vi "Start.vi"(8 "Error In":errorcluster, 11 "Communicator in":refnum<class "Communicator.lvclass">) -> (0 "Error Out":errorcluster, 3 "Communicator out":refnum<class "Communicator.lvclass">)   [LabVIEW 2019, in "Communicator.lvclass"]
uses:
  Communicator.lvclass
  Interfaces/IRunnable/IRunnable.lvclass
  Communicator Worker/Communicator Worker/Communicator Worker.lvclass
  Interfaces/ICommunicate/ICommunicate.lvclass
  Interfaces/IConfigure/IConfigure.lvclass
  Interfaces/IConfiguration/IConfiguration.lvclass
  Communicator.lvclass/Communicator.ctl
  <vilib>/ActorFramework/Actor/Actor.lvclass
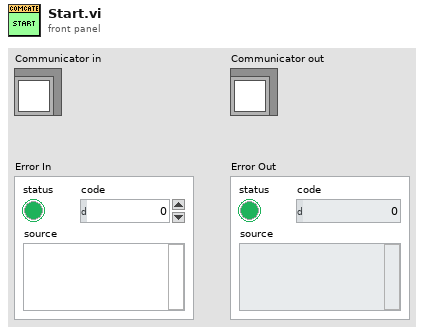
[diagram p1: front panel]
types:
  T1 = typedef "Communicator.lvclass/ObjectAttributes.ctl" = cluster{"IConfigure":refnum<class "IConfigure.lvclass">, "Worker Enqueuer":refnum<class "Message Enqueuer.lvclass">, "Start Counter":i32, "Msg Sent":refnum<user-event>}
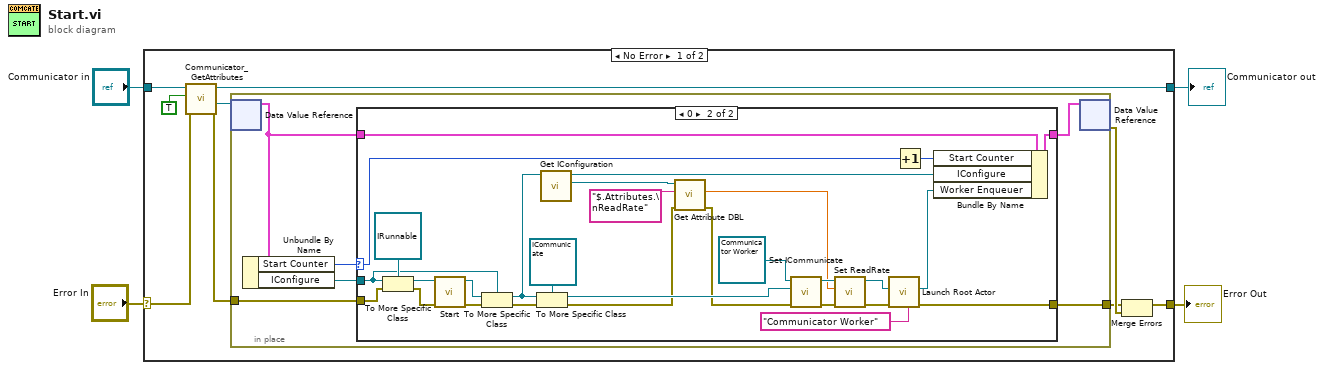
[diagram p0: block diagram]
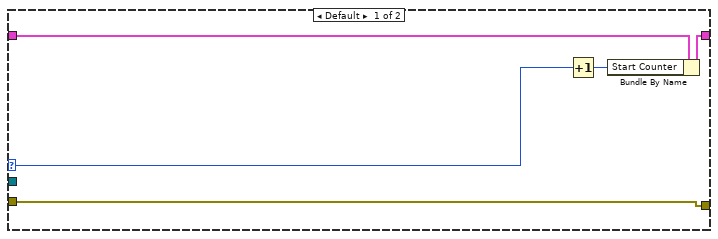
[diagram p2: hidden frame]
diagram:
  n1 = case shown="No Error" "Error In" {
    selector: "Error In" -> [w12 w53]
    tunnel: [w9 w53] -> w3
    tunnel: [w10 w52] -> w1
    tunnel: "Communicator in" -> [w13 w52]
    frame No Error {
      n2 = call "Communicator_GetAttributes.vi"("Error In"=w12, "OnlyGetDvrReference(False)"=TRUE, "Communicator in"=w13) -> ("Error Out"=w6:errorcluster, "DataRef"=w8:refnum<data-value>, "Communicator out"=w10:refnum<class "Communicator.lvclass">)  [unwired: 5 in, 1 out]
      n3 = in-place {
        in-place-border: w6 -> [w17]
        in-place-border: [w16] -> w5
        n4 = in-place-dvr #1(w8) -> (w18:T1)  [unwired: 1 out]
        n5 = Unbundle By Name(w18) -> ("Start Counter"=w14:i32, "IConfigure"=w15:refnum<class "IConfigure.lvclass">)
        n6 = case shown="0" w14 {
          selector: w14 -> [w22 w26]
          tunnel: [w21 w51] -> w19
          tunnel: w18 -> [w23 w50]
          tunnel: w17 -> [w24 w45]
          tunnel: [w24 w44] -> w16
          tunnel: w15 -> [_ w35]
          frame Default {
            n7 = Increment(x=w22) -> (x+1=w20:i32)
            n8 = Bundle By Name(cluster=w23, "Start Counter"=w20) -> (w21:T1)
          }
          frame 0 {
            n9 = To More Specific Class(target class=refnum<class "IRunnable.lvclass"> refnum ("IRunnable.lvclass"), reference=w35, error in=w45) -> (specific class reference=w48:refnum<class "IRunnable.lvclass">, error out=w47:errorcluster)
            n10 = call-dynamic "Start.vi"("error in"=w47, "IRunnable in"=w48) -> ("error out"=w46:errorcluster, "IRunnable out"=w36:refnum<class "IRunnable.lvclass">)  [unwired: 8 in]
            n11 = To More Specific Class(target class=w35, reference=w36, error in=w46) -> (specific class reference=w34:refnum<class "IConfigure.lvclass">, error out=w37:errorcluster)
            n12 = To More Specific Class(target class=refnum<class "ICommunicate.lvclass"> refnum ("ICommunicate.lvclass"), reference=w34, error in=w37) -> (specific class reference=w32:refnum<class "ICommunicate.lvclass">, error out=w29:errorcluster)
            n13 = call-dynamic "Get IConfiguration.vi"("IConfigure in"=w34) -> ("IConfiguration"=w31:refnum<class "IConfiguration.lvclass">, "IConfigure out"=w33:refnum<class "IConfigure.lvclass">)  [unwired: 9 in]
            n14 = call-dynamic "Get Attribute DBL.vi"("error in"=w29, "Attribute"="$.Attributes.\nReadRate", "IConfiguration in"=w31) -> ("error out"=w25:errorcluster, "Value"=w28:dbl)  [unwired: 6 in, 1 out]
            n15 = call "Set ICommunicate.vi"("ICommunicate"=w32, "Worker in"=refnum<class "Communicator Worker.lvclass"> refnum ("Communicator Worker.lvlib:Worker.lvclass")) -> ("Worker out"=w39:refnum<class "Communicator Worker.lvclass">)  [unwired: 9 in]
            n16 = call "Set ReadRate.vi"("ReadRate"=w28, "Worker in"=w39) -> ("Worker out"=w38:refnum<class "Communicator Worker.lvclass">)  [unwired: 9 in]
            n17 = call <vilib>:"Launch Root Actor.vi"("Debug Alias"="Communicator Worker", "error in (no error)"=w25, "Actor"=w38) -> ("error out"=w44:errorcluster, "Actor's Enqueuer"=w42:refnum<class "Message Enqueuer.lvclass">)  [unwired: 7 in]
            n18 = Increment(x=w26) -> (x+1=w27:i32)
            n19 = Bundle By Name(cluster=w50, "Start Counter"=w27, "IConfigure"=w33, "Worker Enqueuer"=w42) -> (w51:T1)
          }
        }
        n20 = in-place-dvr #1(w19) -> (w11:errorcluster)  [unwired: 1 out]
      }
      n21 = Merge Errors(w5, w11) -> (w9:errorcluster)
    }
    frame Error {
    }
  }
  "Error Out" <- w3
  "Communicator out" <- w1
